vi "_ConnectorPaneEditor_SelectShortcutMenu.vi"(8 "error in (no error)":errorcluster, 10 "ItemTag":string, 11 "ConnectorPaneEditor in":refnum<class "_ConnectorPaneEditor.lvclass">) -> (0 "error out":errorcluster, 3 "ConnectorPaneEditor out":refnum<class "_ConnectorPaneEditor.lvclass">)   [LabVIEW 2014, in "_ConnectorPaneEditor.lvclass"]
uses:
  _ConnectorPaneEditor.lvclass
  _ConnectorPaneEditor.lvclass/_ConnectorPaneEditor.ctl
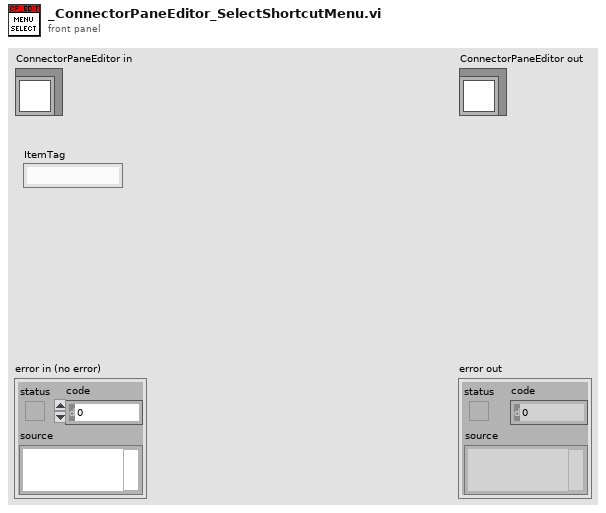
[diagram p1: front panel]
types:
  T1 = enum16{"Invalid Wire Rule", "Required", "Recommended", "Optional", "Dynamic Dispatch"}
  T2 = enum16{"Invalid Wire Rule", "Required", "Recommended", "Optional", "Dynamic Dispatch"}[]
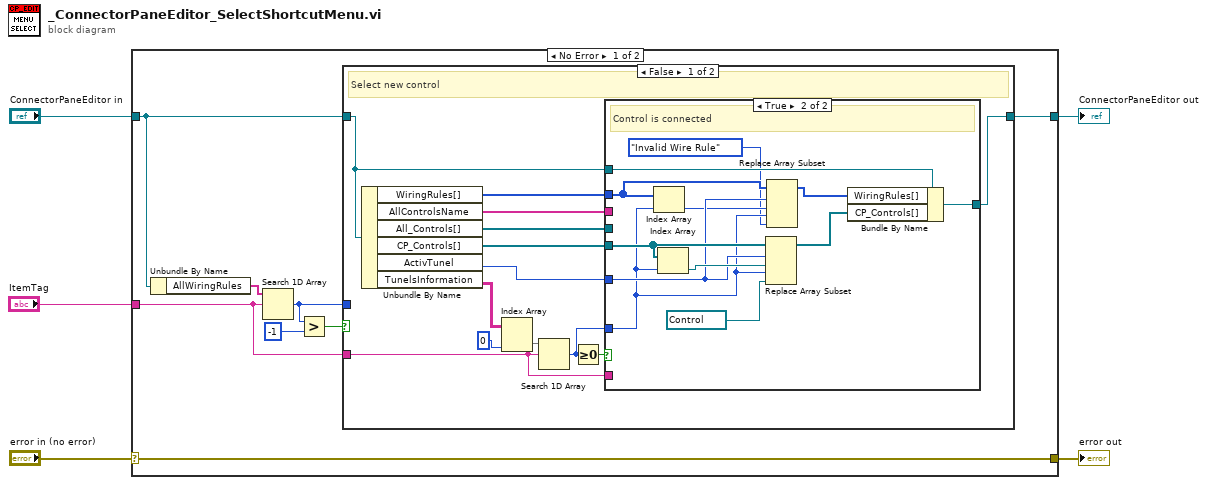
[diagram p0: block diagram]
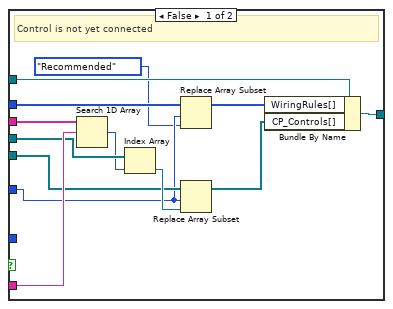
[diagram p2: hidden frame]
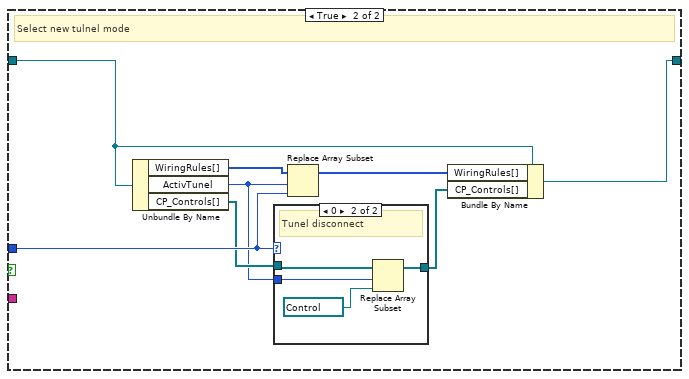
[diagram p3: hidden frame]
diagram:
  n1 = case shown="No Error" "error in (no error)" {
    selector: "error in (no error)" -> [w13 w66]
    tunnel: [w13 w66] -> w4
    tunnel: [w7 w65] -> w2
    tunnel: "ConnectorPaneEditor in" -> [w8 w65]
    tunnel: "ItemTag" -> [w6 _]
    frame No Error {
      n2 = Unbundle By Name(w8) -> ("AllWiringRules"=w12:string[])
      n3 = Search 1D Array(1D array=w12, element=w6) -> (index of element=w9:i32)  [unwired: 1 in]
      n4 = Greater?(x=w9, y=-1) -> (0:w10:bool)
      n5 = case shown="False" w10 {
        tunnel: w8 -> [w18 w58]
        tunnel: w9 -> [_ w55]
        tunnel: [w17 w56] -> w7
        tunnel: w6 -> [w15 _]
        frame False {
          # "Select new control"
          n6 = Unbundle By Name(w18) -> ("WiringRules[]"=w19:T2, "AllControlsName"=w16:string[], "All_Controls[]"=w14:refnum<vi>[], "CP_Controls[]"=w22:refnum<vi>[], "ActivTunel"=w20:u32, "TunelsInformation"=w26:string[][])
          n7 = Index Array(array=w26, index (col)=0 ("disabled index (col)")) -> (element=w24:string[])  [unwired: 1 in]
          n8 = Search 1D Array(1D array=w24, element=w15) -> (index of element=w21:i32)  [unwired: 1 in]
          n9 = Greater Or Equal To 0?(x=w21) -> (x >= 0?=w23:bool)
          n10 = case shown="True" w23 {
            tunnel: w22 -> [w30 w51]
            tunnel: w21 -> [_ w41]
            tunnel: w20 -> [w29 w47]
            tunnel: w19 -> [w31 w48]
            tunnel: w18 -> [w34 w45]
            tunnel: [w33 w44] -> w17
            tunnel: w16 -> [w39 _]
            tunnel: w15 -> [w38 _]
            tunnel: w14 -> [w37 _]
            frame False {
              # "Control is not yet connected"
              n11 = Search 1D Array(1D array=w39, element=w38) -> (index of element=w36:i32)  [unwired: 1 in]
              n12 = Index Array(array=w37, index=w36) -> (element=w35:refnum<vi>)
              n13 = Replace Array Subset(array=w31, new element=T1."Recommended" ("new element/subarray"), index=w29) -> (w27:T2)
              n14 = Replace Array Subset(array=w30, new element=w35, index=w29) -> (w32:refnum<vi>[])
              n15 = Bundle By Name(cluster=w34, "WiringRules[]"=w27, "CP_Controls[]"=w32) -> (w33:refnum<class "_ConnectorPaneEditor.lvclass">)
            }
            frame True {
              # "Control is connected"
              n16 = Index Array(array=w48, index=w41) -> (element=w46:T1)
              n17 = Index Array(array=w51, index=w41) -> (element=w50:refnum<vi>)
              n18 = Replace Array Subset(array=w51, new element #1=w50, index #1=w47, new element #2=refnum<vi> refnum ("Ctl Refnum"), index #2=w41) -> (w42:refnum<vi>[])
              n19 = Replace Array Subset(array=w48, new element #1=w46, index #1=w47, new element #2=T1."Invalid Wire Rule" ("new element/subarray"), index #2=w41) -> (w43:T2)
              n20 = Bundle By Name(cluster=w45, "WiringRules[]"=w43, "CP_Controls[]"=w42) -> (w44:refnum<class "_ConnectorPaneEditor.lvclass">)
            }
          }
        }
        frame True {
          # "Select new tulnel mode"
          n21 = Unbundle By Name(w58) -> ("WiringRules[]"=w59:T2, "ActivTunel"=w52:u32, "CP_Controls[]"=w54:refnum<vi>[])
          n22 = case shown="0" w55 {
            tunnel: w54 -> [w60 w63]
            tunnel: [w60 w64] -> w53
            tunnel: w52 -> [_ w61]
            frame Default {
            }
            frame 0 {
              # "Tunel disconnect"
              n23 = Replace Array Subset(array=w63, new element=refnum<vi> refnum ("Ctl Refnum"), index=w61) -> (w64:refnum<vi>[])
            }
          }
          n24 = Replace Array Subset(array=w59, new element=w55, index=w52) -> (w57:T2)
          n25 = Bundle By Name(cluster=w58, "WiringRules[]"=w57, "CP_Controls[]"=w53) -> (w56:refnum<class "_ConnectorPaneEditor.lvclass">)
        }
      }
    }
    frame Error {
    }
  }
  "error out" <- w4
  "ConnectorPaneEditor out" <- w2
